vi "TagContainer-TestMain.vi"() -> ()   [LabVIEW 2017, in "TagContainer.lvlib"]
uses:
  TagContainer.lvlib
  a1ae43e1-b2e0-48b2-b5bf-09d8c6337ec0.vi
  5d4c14d8-f2b2-4cd0-9f9f-81160b0f88f4.vi
  69a5f5dc-289e-4520-a43d-4a6e53800127.vi
  f6a41f1a-46ba-40d5-b8b9-4f6d9d3cd2d0.vi
  b9594d6d-a8e1-4e69-b527-0d31d87043e6.vi
  _Support/_NameCacher.vi
  _Support/_datatypeChecker.vi
  _Support/_Ref To DVR.vi
  API/TagContainer-ChangeDetector.vi/4615f950-5bb4-4f5c-be7d-266d36556fe4.vi
  <vilib>/Utility/Data Type/Get Type Information.vi
  <vilib>/Utility/error.llb/Trim Whitespace.vi
  <userlib>/_OpenG.lib/comparison/comparison.llb/Variant Changed__ogtk.vi
panel:
  out "TEst":cluster{"Numeric":i32, "String":string}
  out "changed?":bool[](array[boolean])
  in  "Reject New Tag(F)":bool=TRUE
  out "should be datatype error":errorcluster
  out "should be no tag error":errorcluster
  out "Raw name":string
  in  "Type":cluster{"Numeric":i32, "String":string}
  in  "Stop":bool
  out "Value":cluster{"Numeric":i32, "String":string}
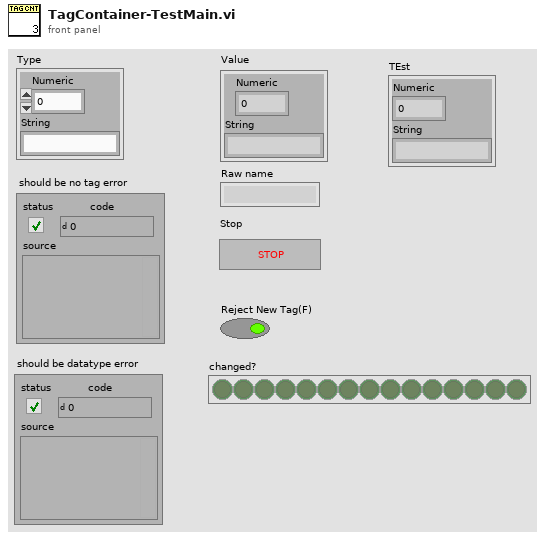
[diagram p1: front panel]
types:
  T1 = typedef "TagContainer.lvlib/TagContainer.ctl" = refnum<k1>
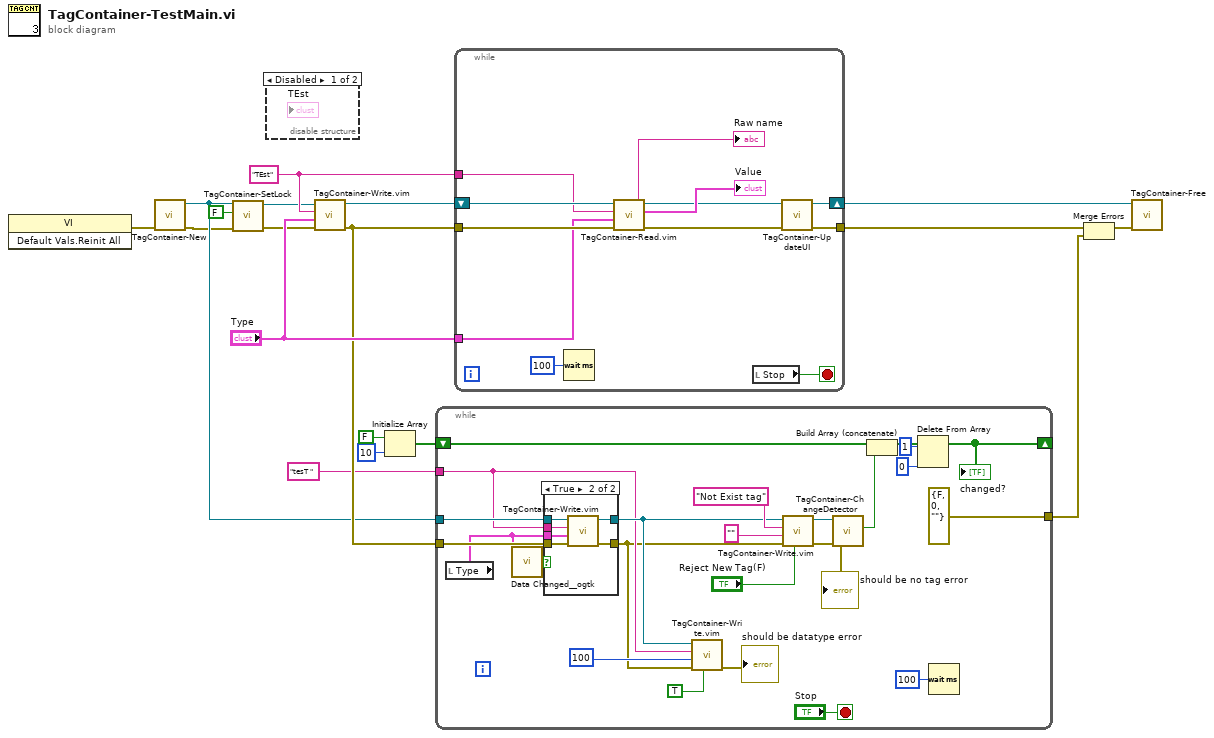
[diagram p0: block diagram]
diagram:
  w14 = "TEst" ("name")
  n1 = invoke class="VI" method="Default Vals.Reinit All"() -> (error out=w10:errorcluster)  [unwired: 3 in, 2 out]
  n2 = call "TagContainer-New.vi"("error in (no error)"=w10) -> ("error out"=w4:errorcluster, "TagContainer"=w5:T1)  [unwired: 9 in]
  n3 = call "TagContainer-SetLock.vi"("error in (no error)"=w4, "Lock?(T)"=FALSE, "TagContainer"=w5) -> ("error out"=w3:errorcluster, "TagContainer(dup)"=w2:T1)  [unwired: 7 in]
  n4 = disable-structure shown="Disabled" {
    frame Disabled {
    }
    frame Enabled {
    }
  }
  n5 = call "TagContainer-Write.vim"("error in (no error)"=w3, "Value"="Type", "name"=w14, "TagContainer"=w2) -> ("error out"=w13:errorcluster, "TagContainer(dup)"=w18:T1)  [unwired: 6 in]
  n6 = Initialize Array(FALSE, 10 ("dimension size")) -> (w6:bool[])
  n7 = while {
    tunnel: w5 -> [w40]
    tunnel: "tesT " ("name") -> [w32]
    tunnel: w13 -> [w39]
    tunnel: [errorcluster {"status"=FALSE, "code"=0, "source"=""} ("error out")] -> w11
    shift-right: [w23] -> _
    shift-left: w6 -> [w26]
    stop <- "Stop" stop-if-true
    n8 = local read "Type"() -> (w20:cluster{"Numeric":i32, "String":string})
    n9 = call-poly <userlib>:"Data Changed__ogtk.vi"("Variant"=w20) -> ("Changed"=w19:bool)
    n10 = case shown="True" w19 {
      tunnel: w40 -> [w44 w50]
      tunnel: w39 -> [w43 w49]
      tunnel: [w44 w48] -> w33
      tunnel: w32 -> [_ w47]
      tunnel: [w43 w46] -> w30
      tunnel: w20 -> [_ w45]
      frame False {
      }
      frame True {
        n11 = call "TagContainer-Write.vim"("error in (no error)"=w49, "Value"=w45, "name"=w47, "TagContainer"=w50) -> ("error out"=w46:errorcluster, "TagContainer(dup)"=w48:T1)  [unwired: 6 in]
      }
    }
    n12 = call "TagContainer-Write.vim"("Reject New Tag(F)"=TRUE, "error in (no error)"=w30, "Value"=u32 100 ("milliseconds to wait"), "name"=w32, "TagContainer"=w33) -> ("error out"=→"should be datatype error":errorcluster)  [unwired: 5 in, 1 out]
    n13 = call "TagContainer-Write.vim"("Reject New Tag(F)"="Reject New Tag(F)", "error in (no error)"=w30, "Value"="" ("name"), "name"="Not Exist tag", "TagContainer"=w33) -> ("error out"=→"should be no tag error":errorcluster, "TagContainer(dup)"=w27:T1)  [unwired: 5 in]
    n14 = call "TagContainer-ChangeDetector.vi"("TagContainer"=w27) -> ("Changed"=w25:bool)  [unwired: 8 in, 2 out]
    n15 = Build Array (concatenate)(w26, w25) -> (w24:bool[])
    n16 = Delete From Array(array=w24, length=1, index=0) -> (array with subset deleted=w23:bool[])  [unwired: 1 out]
    "changed?" <- w23
    n17 = Wait (ms)(milliseconds to wait=u32 100) -> ()  [unwired: 1 out]
  }
  n18 = while {
    tunnel: w14 -> [w60]
    tunnel: "Type" -> [w59]
    shift-right: [w51] -> w17
    shift-left: w18 -> [w62]
    tunnel: w13 -> [w61]
    tunnel: [w52] -> w16
    stop <- w57 stop-if-true
    n19 = Wait (ms)(milliseconds to wait=u32 100) -> ()  [unwired: 1 out]
    n20 = call "TagContainer-Read.vim"("error in (no error)"=w61, "Type"=w59, "name"=w60, "TagContainer"=w62) -> ("error out"=w53:errorcluster, "Value"=→"Value":cluster{"Numeric":i32, "String":string}, "TagContainer(dup)"=w54:T1, "Raw name"=→"Raw name":string)  [unwired: 2 in, 2 out]
    n21 = local read "Stop"() -> (w57:bool)
    n22 = call "TagContainer-UpdateUI.vi"("error in (no error)"=w53, "TagContainer"=w54) -> ("error out"=w52:errorcluster, "TagContainer(dup)"=w51:T1)  [unwired: 8 in]
  }
  n23 = Merge Errors(w16, w11) -> (w12:errorcluster)
  n24 = call "TagContainer-Free.vi"("error in (no error)"=w12, "TagContainer"=w17) -> ()  [unwired: 9 in, 1 out]
